vi "实验2_2.vi"() -> ()   [LabVIEW 2018]
panel:
  out "output":dbl(graph)
  in  "?":bool
  out "?":dbl
  in  "delay":u32(slide) scale=0.0..500.0
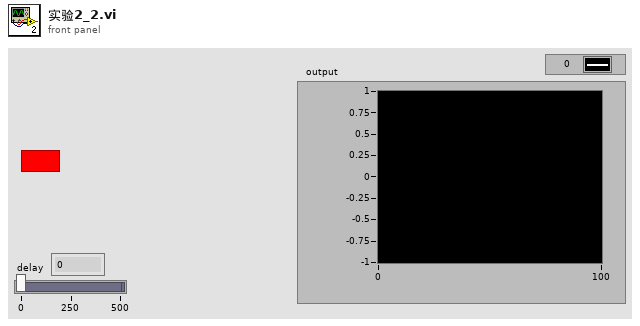
[diagram p1: front panel]
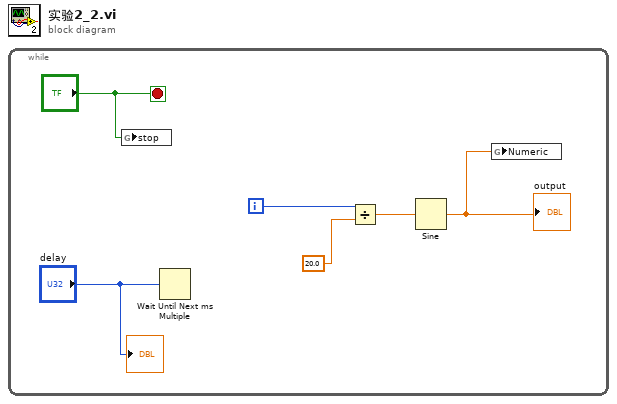
[diagram p0: block diagram]
diagram:
  n1 = while {
    i -> [w5]
    stop <- "?" stop-if-true
    n2 = global write "实验2_2全局.vi" "stop"("?") -> ()
    n3 = Wait Until Next ms Multiple(millisecond multiple="delay") -> ()  [unwired: 1 out]
    n4 = Divide(x=w5, y=20.0) -> (x/y=w3:dbl)
    n5 = Sine ("正弦")(x=w3) -> (sin(x)=w2:dbl)
    "output" <- w2
    n6 = global write "实验2_2全局.vi" "Numeric"(w2) -> ()
    "?" <- "delay"
  }
